vi "Filter_for_tree.vi"(5 "Ch Name":string, 7 "Tolerance":dbl=1.0 format="%.2f", 8 "Precision":i32, 9 "Ch Values In":string[](array[string])) -> (1 "Accept array":bool[][](array[boolean]), 2 "Bin Names":string[](array[string]))   [LabVIEW 2010]
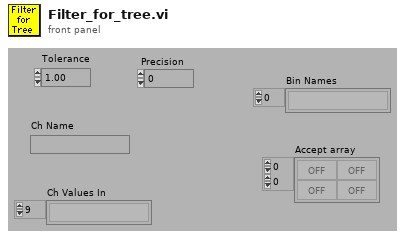
[diagram p1: front panel]
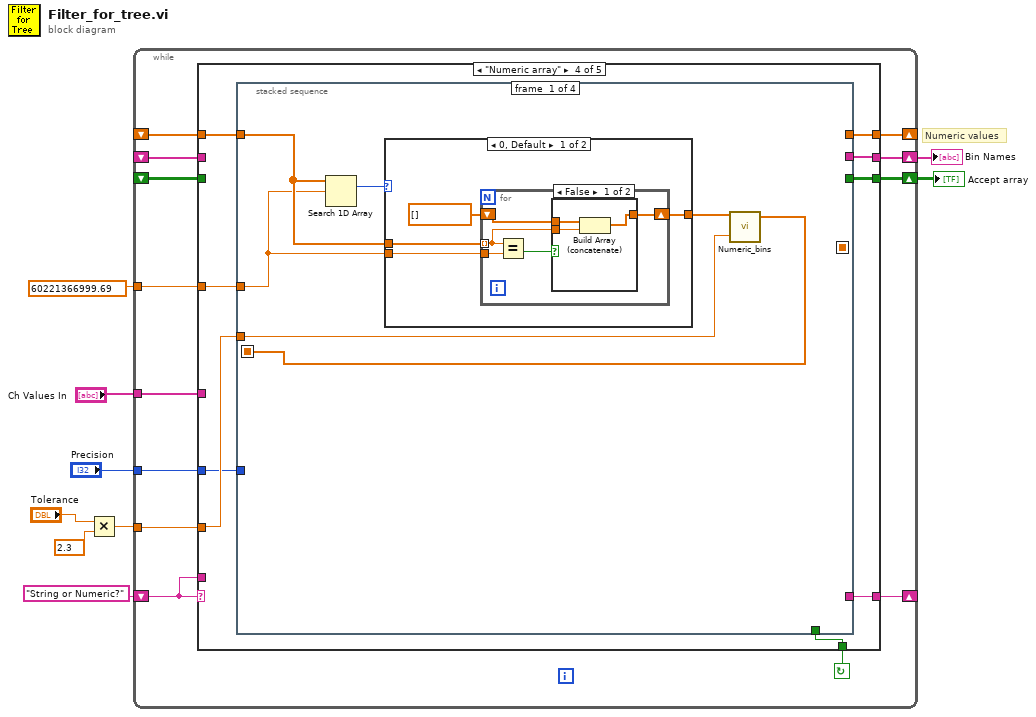
[diagram p0: block diagram]
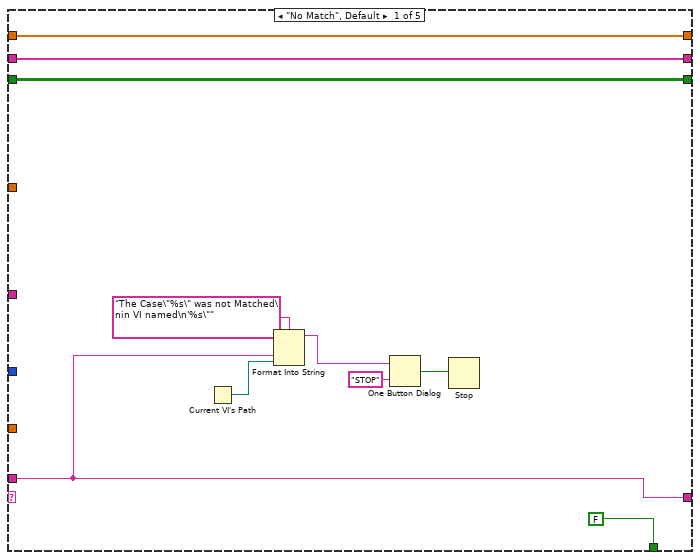
[diagram p2: hidden frame]
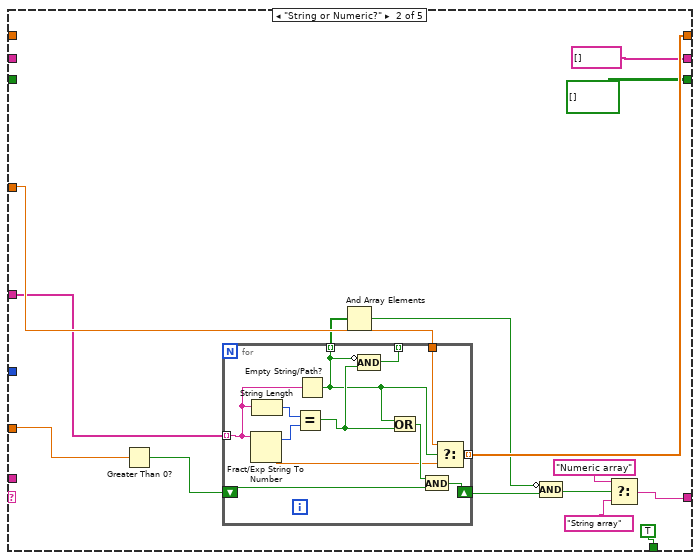
[diagram p3: hidden frame]
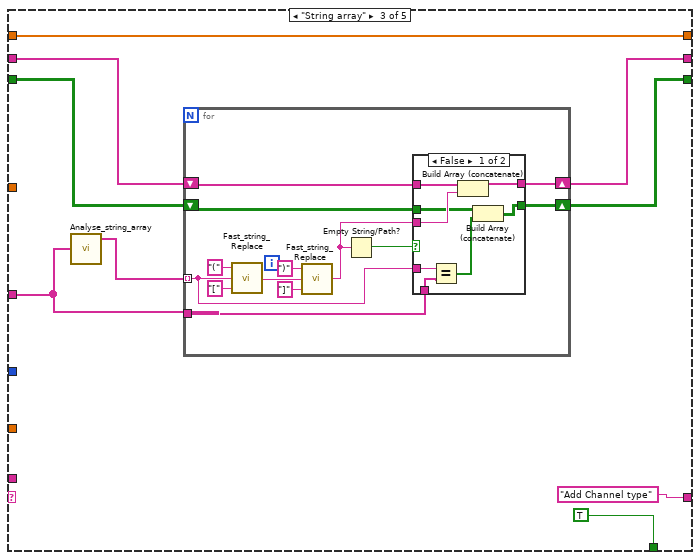
[diagram p4: hidden frame]
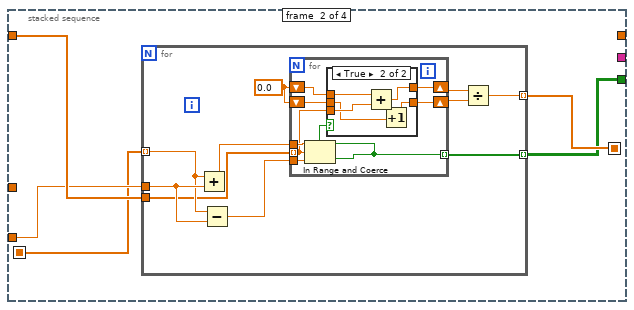
[diagram p8: hidden frame]
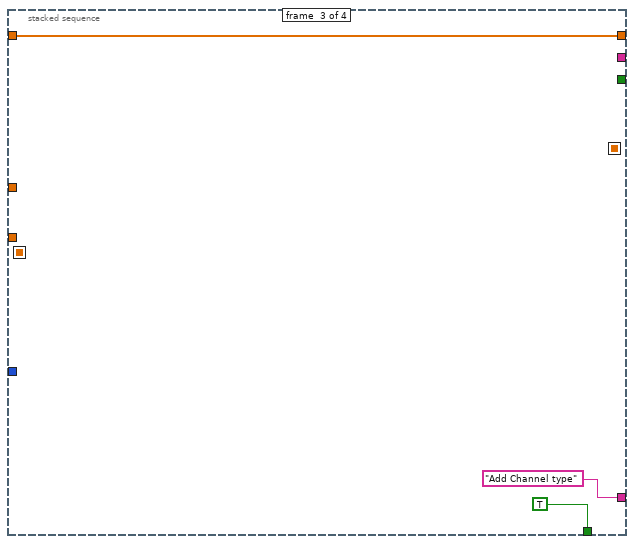
[diagram p10: hidden frame]
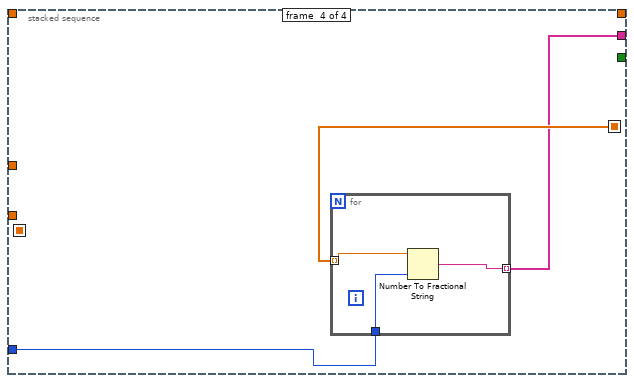
[diagram p11: hidden frame]
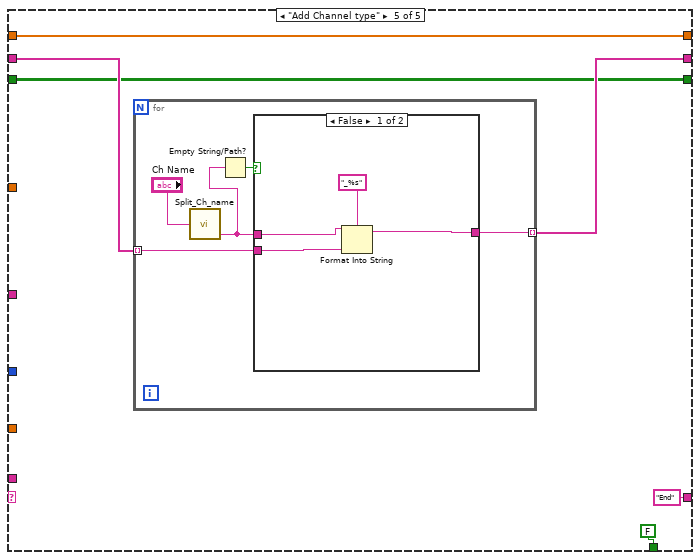
[diagram p12: hidden frame]
diagram:
  # "Numeric values"
  n1 = Multiply(x="Tolerance", y=2.3) -> (x*y=w2:dbl)
  n2 = while {
    tunnel: "Precision" -> [w10]
    shift-left: _ -> [w11]
    shift-right: [w12] -> w5
    shift-left: _ -> [w13]
    shift-right: [w14] -> w6
    tunnel: "Ch Values In" -> [w15]
    tunnel: w2 -> [w16]
    shift-left: _ -> [w17]
    shift-right: [w21] -> _
    shift-left: "String or Numeric?" -> [w18]
    shift-right: [w20] -> _
    tunnel: 60221366999.69 ("number") -> [w22]
    stop <- w19 continue-if-true
    n3 = case shown="\"Numeric array\"" w18 {
      tunnel: w22 -> [_ w40 _ w95 _]
      tunnel: [w31 w47 w67 w97 w165] -> w21
      tunnel: [w25 w44 "Add Channel type" w99 "End"] -> w20
      tunnel: [FALSE TRUE TRUE w100 FALSE] -> w19
      tunnel: w18 -> [w25 _ _ _ _]
      tunnel: w17 -> [w31 _ w67 w96 w165]
      tunnel: w16 -> [_ w43 _ w98 _]
      tunnel: w15 -> [_ w36 w64 _ _]
      tunnel: [w24 string[] [] w63 w94 w163] -> w14
      tunnel: w13 -> [w24 _ w62 _ w164]
      tunnel: [w23 bool[][] [] w60 w93 w162] -> w12
      tunnel: w11 -> [w23 _ w61 _ w162]
      tunnel: w10 -> [_ _ _ w92 _]
      frame "No Match", Default {
        n4 = Current VI's Path() -> (path=w26:path)
        n5 = Format Into String(format string="The Case\"%s\" was not Matched\nin VI named\n'%s\"" ("Format String"), w25, w26) -> (resulting string=w29:string)  [unwired: 2 in, 1 out]
        n6 = One Button Dialog(message=w29, button name ("OK")="STOP") -> (true=w27:bool)
        n7 = Stop(stop? (T)=w27) -> ()
      }
      frame "String or Numeric?" {
        n8 = Greater Than 0?(x=w43) -> (x > 0?=w42:bool)
        n9 = for {
          tunnel: w36 -> [w52] mode=indexing
          shift-right: [w57] -> w39
          shift-left: w42 -> [w58]
          tunnel: [w56] -> w47 mode=indexing
          tunnel: [w50] -> w35 mode=indexing
          tunnel: w40 -> [w49]
          tunnel: [w48] -> _ mode=indexing
          n10 = Fract/Exp String To Number(string=w52) -> (offset past number=w54:i32, number=w55:dbl)  [unwired: 3 out]
          n11 = String Length(string=w52) -> (length=w53:i32)
          n12 = Equal?(x=w53, y=w54) -> (x = y?=w51:bool)
          n13 = Empty String/Path?(string/path=w52) -> (empty?=w50:bool)
          n14 = Compound Arithmetic op=AND(invert w50, w51) -> (w48:bool)
          n15 = Or(x=w50, y=w51) -> (x .or. y?=w59:bool)
          n16 = And(x=w59, y=w58) -> (x .and. y?=w57:bool)
          n17 = Select(t=w49, s=w50, f=w55) -> (s? t:f=w56:dbl)
        }
        n18 = And Array Elements(Boolean array=w35) -> (logical AND=w38:bool)
        n19 = Compound Arithmetic op=AND(invert w38, w39) -> (w37:bool)
        n20 = Select(t="Numeric array", s=w37, f="String array") -> (s? t:f=w44:string)
      }
      frame "String array" {
        n21 = call "Analyse_string_array.vi"("String array"=w64) -> ("Unique strings"=w65:string[])  [unwired: 2 out]
        n22 = for {
          tunnel: w64 -> [w69]
          tunnel: w65 -> [w70] mode=indexing
          shift-right: [w74] -> w63
          shift-left: w62 -> [w75]
          shift-right: [w71] -> w60
          shift-left: w61 -> [w72]
          n23 = call "Fast_string_Replace.vi"("Replace match with:"="[", "Input String"=w70, "regular expression"="(") -> ("Output String"=w77:string)  [unwired: 2 out]
          n24 = call "Fast_string_Replace.vi"("Replace match with:"="]", "Input String"=w77, "regular expression"=")") -> ("Output String"=w73:string)  [unwired: 2 out]
          n25 = Empty String/Path?(string/path=w73) -> (empty?=w76:bool)
          n26 = case shown="False" w76 {
            tunnel: w75 -> [w89 w91]
            tunnel: [w88 w91] -> w74
            tunnel: w73 -> [w87 _]
            tunnel: w72 -> [w86 w90]
            tunnel: [w85 w90] -> w71
            tunnel: w70 -> [w84 _]
            tunnel: w69 -> [w83 _]
            frame False {
              n27 = Equal?(x=w84, y=w83) -> (x = y?=w82:bool[])
              n28 = Build Array (concatenate)(w89, w87) -> (w88:string[])
              n29 = Build Array (concatenate)(w86, w82) -> (w85:bool[][])
            }
            frame True {
            }
          }
        }
      }
      frame "Numeric array" {
        n30 = stacked-sequence {
          seq-local: [_ w122 _ _] -> [_ _ _ w156]
          seq-local: [w101 _ _ _] -> [_ w123 _ _]
          tunnel: w98 -> [w104 w124 _ _]
          tunnel: [_ _ w151 _] -> w97
          tunnel: w96 -> [w106 w125 w151 _]
          tunnel: [_ _ TRUE _] -> w100
          tunnel: [_ _ "Add Channel type" _] -> w99
          tunnel: w95 -> [w102 _ _ _]
          tunnel: [_ _ _ w155] -> w94
          tunnel: [_ w121 _ _] -> w93
          tunnel: w92 -> [_ _ _ w154]
          frame #0 {
            n31 = Search 1D Array(1D array=w106, element=w102) -> (index of element=w103:i32)  [unwired: 1 out]
            n32 = case shown="0, Default" w103 {
              tunnel: w106 -> [w110 w120]
              tunnel: w102 -> [w109 _]
              tunnel: [w107 w120] -> w105
              frame 0, Default {
                n33 = for {
                  shift-right: [w113] -> w107
                  shift-left: dbl[] [] -> [w114]
                  tunnel: w110 -> [w111] mode=indexing
                  tunnel: w109 -> [w112]
                  n34 = Equal?(x=w111, y=w112) -> (x = y?=w115:bool)
                  n35 = case shown="False" w115 {
                    tunnel: w114 -> [w118 w119]
                    tunnel: [w117 w119] -> w113
                    tunnel: w111 -> [w116 _]
                    frame False {
                      n36 = Build Array (concatenate)(w118, w116) -> (w117:dbl[])
                    }
                    frame True {
                    }
                  }
                }
              }
              frame -1 {
              }
            }
            n37 = call "Numeric_bins.vi"("Values"=w105, "Tolerance"=w104) -> ("Bin Centres"=w101:dbl[])  [unwired: 2 out]
          }
          frame #1 {
            n38 = for {
              tunnel: w123 -> [w133] mode=indexing
              tunnel: w124 -> [w135]
              tunnel: w125 -> [w128]
              tunnel: [w127] -> w121 mode=indexing
              tunnel: [w126] -> w122 mode=indexing
              w130 = 0.0
              n39 = Add(x=w133, y=w135) -> (x+y=w129:dbl)
              n40 = Subtract(x=w133, y=w135) -> (x-y=w134:dbl)
              n41 = for {
                tunnel: w129 -> [w143]
                tunnel: w134 -> [w142]
                tunnel: w128 -> [w138] mode=indexing
                tunnel: [w141] -> w127 mode=indexing
                shift-right: [w139] -> w132
                shift-left: w130 -> [w140]
                shift-right: [w136] -> w131
                shift-left: w130 -> [w137]
                n42 = In Range and Coerce(upper limit=w143, x=w138, lower limit=w142) -> (In Range?=w141:bool)  [unwired: 1 out]
                n43 = case shown="True" w141 {
                  tunnel: w140 -> [w145 w150]
                  tunnel: [w145 w149] -> w139
                  tunnel: w138 -> [_ w148]
                  tunnel: w137 -> [w144 w146]
                  tunnel: [w144 w147] -> w136
                  frame False {
                  }
                  frame True {
                    n44 = Add(x=w150, y=w148) -> (x+y=w149:dbl)
                    n45 = Increment(x=w146) -> (x+1=w147:dbl)
                  }
                }
              }
              n46 = Divide(x=w132, y=w131) -> (x/y=w126:dbl)
            }
          }
          frame #2 {
          }
          frame #3 {
            n47 = for {
              tunnel: w156 -> [w158] mode=indexing
              tunnel: [w157] -> w155 mode=indexing
              tunnel: w154 -> [w159]
              n48 = Number To Fractional String(number=w158, precision (6)=w159) -> (F-format string=w157:string)  [unwired: 2 out]
            }
          }
        }
      }
      frame "Add Channel type" {
        n49 = for {
          tunnel: w164 -> [w170] mode=indexing
          tunnel: [w169] -> w163 mode=indexing
          n50 = call "Split_Ch_name.vi"("Ch name"="Ch Name") -> ("Low level"=w167:string)  [unwired: 2 out]
          n51 = Empty String/Path?(string/path=w167) -> (empty?=w166:bool)
          n52 = case shown="False" w166 {
            tunnel: w170 -> [w174 w175]
            tunnel: [w173 w175] -> w169
            tunnel: w167 -> [w171 _]
            frame False {
              n53 = Format Into String(format string="_%s" ("Format String"), initial string=w171, w174) -> (resulting string=w173:string)  [unwired: 1 in, 1 out]
            }
            frame True {
            }
          }
        }
      }
    }
  }
  "Bin Names" <- w6
  "Accept array" <- w5
